vi "STN neuron.vi"(4 "In 6":bool, 6 "In 5":bool, 8 "In 4":bool, 9 "In 3":bool, 10 "In 2":bool, 11 "In":bool) -> (3 "Out":bool)   [LabVIEW 2014]
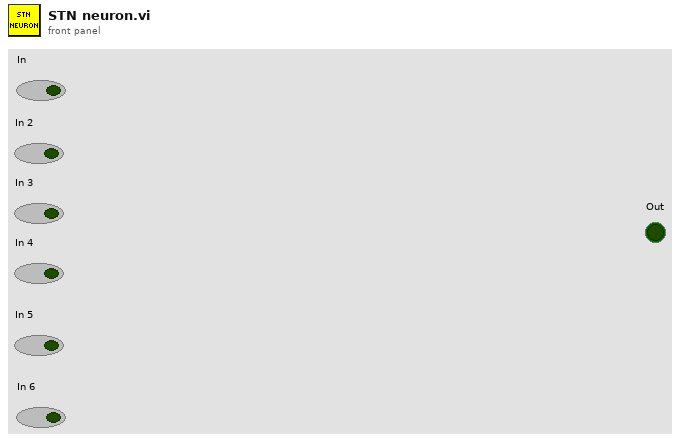
[diagram p1: front panel]
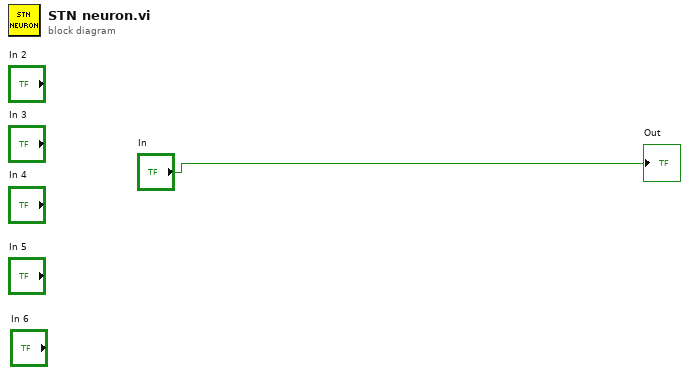
[diagram p0: block diagram]
diagram:
  "Out" <- "In"
